vi "POSITION ARMS MANUAL TELEOP.vi"(11 "Joystick values":T1(array[cluster])) -> ()   [LabVIEW 2020]
uses:
  <vilib>/Rock Robotics/Network Tables/NT Read Number.vi
  <vilib>/Rock Robotics/Network Tables/NT Write Number.vi
  Robot Global Data.vi
  <vilib>/Rock Robotics/Network Tables/NT Read Boolean.vi
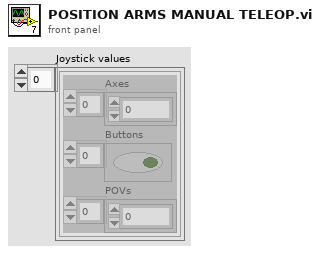
[diagram p1: front panel]
types:
  T1 = cluster{"Axes":dbl[], "Buttons":bool[], "POVs":i16[]}[]
  T2 = cluster{"Axes":dbl[], "Buttons":bool[], "POVs":i16[]}
  T3 = cluster{"MIN":dbl, "MAX":dbl, "convert climber inches to tics":dbl}
  T4 = cluster{"MIN":dbl, "MAX":dbl, "convert arm inches to revs":dbl}
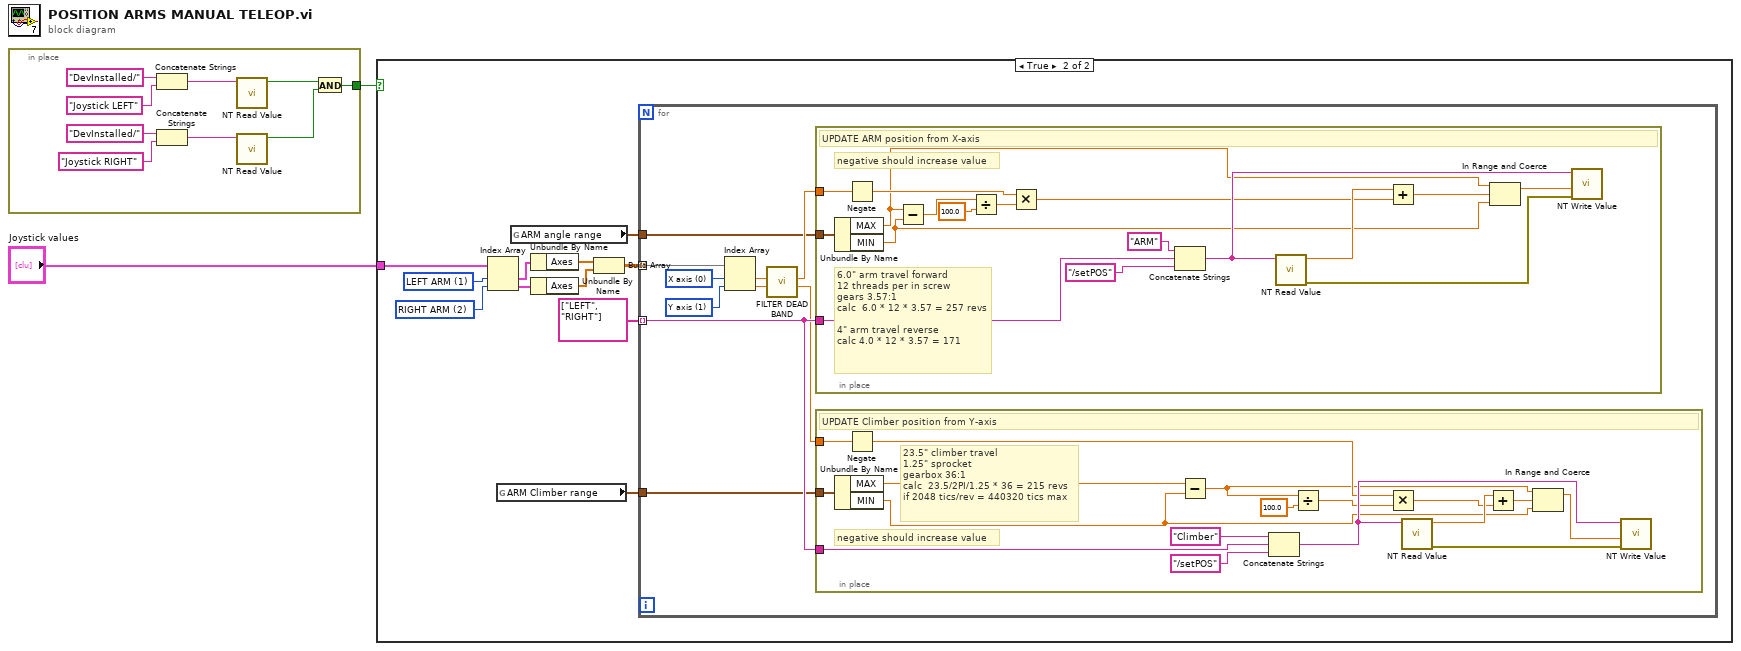
[diagram p0: block diagram]
diagram:
  n1 = in-place {
    in-place-border: [w3] -> w1
    n2 = Concatenate Strings("DevInstalled/" ("Name"), "Joystick LEFT" ("Name")) -> (w11:string)
    n3 = Concatenate Strings("DevInstalled/" ("Name"), "Joystick RIGHT" ("Name")) -> (w8:string)
    n4 = call-poly <vilib>:"NT Read Value.vi"("Name"=w11) -> ("Boolean"=w4:bool)  [unwired: 9 in, 1 out]
    n5 = call-poly <vilib>:"NT Read Value.vi"("Name"=w8) -> ("Boolean"=w5:bool)  [unwired: 9 in, 1 out]
    n6 = And(x=w4, y=w5) -> (x .and. y?=w3:bool)
  }
  n7 = case shown="True" w1 {
    tunnel: "Joystick values" -> [_ w18]
    frame False {
    }
    frame True {
      w14 = u16 2 items=["RIGHT TANK (default)", "LEFT ARM", "RIGHT ARM", "LEFT TANK DRIVE"] ("Joysticks")
      w19 = u16 1 items=["RIGHT TANK (default)", "LEFT ARM", "RIGHT ARM", "LEFT TANK DRIVE"] ("Joysticks")
      n8 = Index Array(array=w18, index #1=w19, index #2=w14) -> (element #1=w17:T2, element #2=w13:T2)
      n9 = global read "Robot Global Data.vi" "ARM Climber range"() -> (w21:T3)
      n10 = global read "Robot Global Data.vi" "ARM angle range"() -> (w20:T4)
      n11 = Unbundle By Name(w17) -> ("Axes"=w15:dbl[])
      n12 = Unbundle By Name(w13) -> ("Axes"=w12:dbl[])
      n13 = Build Array(w15, w12) -> (w16:dbl[][])
      n14 = for {
        tunnel: string[] ["LEFT", "RIGHT"] -> [w28] mode=indexing
        tunnel: w16 -> [w32] mode=indexing
        tunnel: w21 -> [w26]
        tunnel: w20 -> [w25]
        w23 = u16 1 items=["X axis", "Y axis", "Z axis"] ("AXIS VALUES")
        w24 = u16 0 items=["X axis", "Y axis", "Z axis"] ("AXIS VALUES")
        n15 = Index Array(array=w32, index #1=w24, index #2=w23) -> (element #1=w31:dbl, element #2=w30:dbl)
        n16 = call "FILTER DEAD BAND.vi"("Joystick value in 2"=w30, "Joystick value in"=w31) -> ("Joystick value out 2"=w27:dbl, "Joystick value out"=w29:dbl)  [unwired: 8 in]
        n17 = in-place {
          in-place-border: w28 -> [w66]
          in-place-border: w29 -> [w58]
          in-place-border: w25 -> [w52]
          # "6.0\" arm travel forward\n12 threads per in screw\ngears 3.57:1\ncalc  6.0 * 12 * 3.57 = 257 revs\n\n4\" arm travel reverse\ncalc 4.0 * 12 * 3.57 = 171"
          # "negative should increase value"
          # "UPDATE ARM position from X-axis"
          n18 = Unbundle By Name(w52) -> ("MAX"=w51:dbl, "MIN"=w50:dbl)
          n19 = Negate(x=w58) -> (-x=w57:dbl)
          n20 = Subtract(x=w51, y=w50) -> (x-y=w53:dbl)
          n21 = Divide(x=w53, y=100.0) -> (x/y=w55:dbl)
          n22 = Multiply(x=w57, y=w55) -> (x*y=w59:dbl)
          n23 = Concatenate Strings("ARM" ("string"), w66, "/setPOS" ("string")) -> (w62:string)
          n24 = call-poly <vilib>:"NT Read Value.vi"("Name"=w62) -> ("error out"=w63:errorcluster, "Numeric"=w60:dbl)  [unwired: 9 in]
          n25 = Add(x=w60, y=w59) -> (x+y=w61:dbl)
          n26 = In Range and Coerce(upper limit=w51, x=w61, lower limit=w50) -> (coerced(x)=w56:dbl)  [unwired: 1 out]
          n27 = call-poly <vilib>:"NT Write Value.vi"("error in"=w63, "Numeric"=w56, "Name"=w62) -> ()  [unwired: 8 in, 1 out]
        }
        n28 = in-place {
          in-place-border: w28 -> [w49]
          in-place-border: w27 -> [w41]
          in-place-border: w26 -> [w36]
          # "23.5\" climber travel\n1.25\" sprocket\ngearbox 36:1\ncalc  23.5/2PI/1.25 * 36 = 215 revs\nif 2048 tics/rev = 440320 tics max"
          # "negative should increase value"
          # "UPDATE Climber position from Y-axis"
          n29 = Unbundle By Name(w36) -> ("MAX"=w35:dbl, "MIN"=w33:dbl)
          n30 = Negate(x=w41) -> (-x=w40:dbl)
          n31 = Subtract(x=w35, y=w33) -> (x-y=w34:dbl)
          n32 = Concatenate Strings("Climber" ("string"), w49, "/setPOS" ("string")) -> (w45:string)
          n33 = Divide(x=w34, y=100.0) -> (x/y=w38:dbl)
          n34 = Multiply(x=w40, y=w38) -> (x*y=w42:dbl)
          n35 = call-poly <vilib>:"NT Read Value.vi"("Name"=w45) -> ("error out"=w46:errorcluster, "Numeric"=w43:dbl)  [unwired: 9 in]
          n36 = Add(x=w43, y=w42) -> (x+y=w44:dbl)
          n37 = In Range and Coerce(upper limit=w34, x=w44, lower limit=w33) -> (coerced(x)=w39:dbl)  [unwired: 1 out]
          n38 = call-poly <vilib>:"NT Write Value.vi"("error in"=w46, "Numeric"=w39, "Name"=w45) -> ()  [unwired: 8 in, 1 out]
        }
      }
    }
  }
